vi "FormCalibra10-joao.vi"() -> ()   [LabVIEW 2014]
uses:
  testMachine.ctl
  mainMachine.ctl
  <vilib>/Instr/_visa.llb/VISA Configure Serial Port (Instr).vi
  <vilib>/express/express shared/transition.llb/Dynamic To Waveform Array.vi
  <vilib>/express/express signal manip/GetorSetDDTAttributes/Set DDT Attributes/SetT0.vi
  <vilib>/express/express shared/transition.llb/Waveform Array To Dynamic.vi
  <vilib>/express/express signal manip/GetorSetDDTAttributes/Set DDT Attributes/Set DDT Properties.xnode
panel:
  in  "editSpeedOffset":dbl caption="Offset (Km/h)"
  in  "editSetTempRefB":dbl caption="Offset B" step=0.01 format="%#_2f"
  in  "VISA Serial Port":refnum<visa-resource-name>
  in  "Lower level":dbl
  in  "hysteresis":dbl format="%.2p"
  in  "level":dbl format="%.2p"
  out "rpm":bool
  out "editTotalWaitLimit":u8
  out "editCountWaitLimit":u8
  out "ledWaitState":bool caption="Wait State"
  out "sliderWaitUpperTime":u8(slide) max=50 scale=0.0..100.0
  out "slideWaitLowerTime":u8(slide) max=30 scale=0.0..100.0
  out "slideWaitTime":u8(slide) scale=0.0..100.0
  out "labelTestTime":string caption="Tempo total de ensaio"
  in  "editSetWaitTime":u8 caption="Interval between snubs (s)" step=1 format="%0d"
  in  "stop":bool
  out "ledAcquireState":bool caption="Acquire State"
  out "editTotalLowerLimit":u8
  out "editCountLowerLimit":u8
  out "editTotalUpperLimit":u8
  out "editCountUpperLimit":u8
  out "ledEnsaio 3":bool
  out "ledBrakeState":bool caption="Brake State"
  out "ledExitState":bool caption="Exit State"
  out "ledMotorState":bool caption="Motor State"
  out "ledInit2State":bool caption="Init State"
  out "ledBlockState":bool caption="Block State"
  out "ledRunningState":bool caption="Running State"
  out "ledReadyState":bool caption="Ready State"
  out "ledInitState":bool caption="Init State"
  out "mainMachine":T1
  out "testMachine":T2=enum."finish"
  in  "editSetPathToFile":path
  in  "buttonStop":bool
  in  "buttonStart":bool
  out "graphForce":dynamicdata(graph)
  in  "editOffsetForce":dbl caption="Tare (KN)" min=-100.0 max=100.0 step=0.1
  in  "editSetForce":dbl=0.1 caption="Conversion Factor" min=0.1 max=100.0 step=0.1
  out "editForce":dbl caption="Force (KN)" format="%#_4f"
  out "graphSpeed":dynamicdata(graph)
  in  "editSetSpeed":dbl caption="Conversion Factor"
  out "editSpeed":dbl caption="Speed (km/h)" format="%#_4f"
  out "editEngineSpeed":dbl caption="Frequency (Hz)" format="%#_4f"
  in  "editSetWaitLowerTime":u8 caption="Lower Wait Interval (s)"
  in  "editSetWaitUpperTime":u8=3 caption="Upper Wait Interval (s)"
  in  "editSetNumberOfCycles":u16 caption="Number of snubs" max=999 step=1 format="%0d"
  in  "editSetLowerLimit":u32 caption="Lower Limit (km/h)"
  in  "editSetUpperLimit":u32 caption="Upper Limit (km/h)"
  out "editTempB":dbl caption="Temperature B (ºC)"
  out "editTempA":dbl caption="Temperature A (ºC)"
  in  "editSetTempRefA":dbl caption="Offset A" step=0.01 format="%#_2f"
  out "ledMotor":bool
  out "ledBrake":bool
  out "ledEnsaio":bool
  out "labelTotalCycle":string
  out "labelCurrentCycle":string
  out "labelSystemTitle":string
  in  "editCurrCycleCtr":u32
  in  "velocidade 2":u32
  out "velocidade":u32
  # "Brake Test Bench"
  # "Com Port"
  # "Temperature"
  # "Rotation"
  # "Load Cell"
  # "Test Configuration"
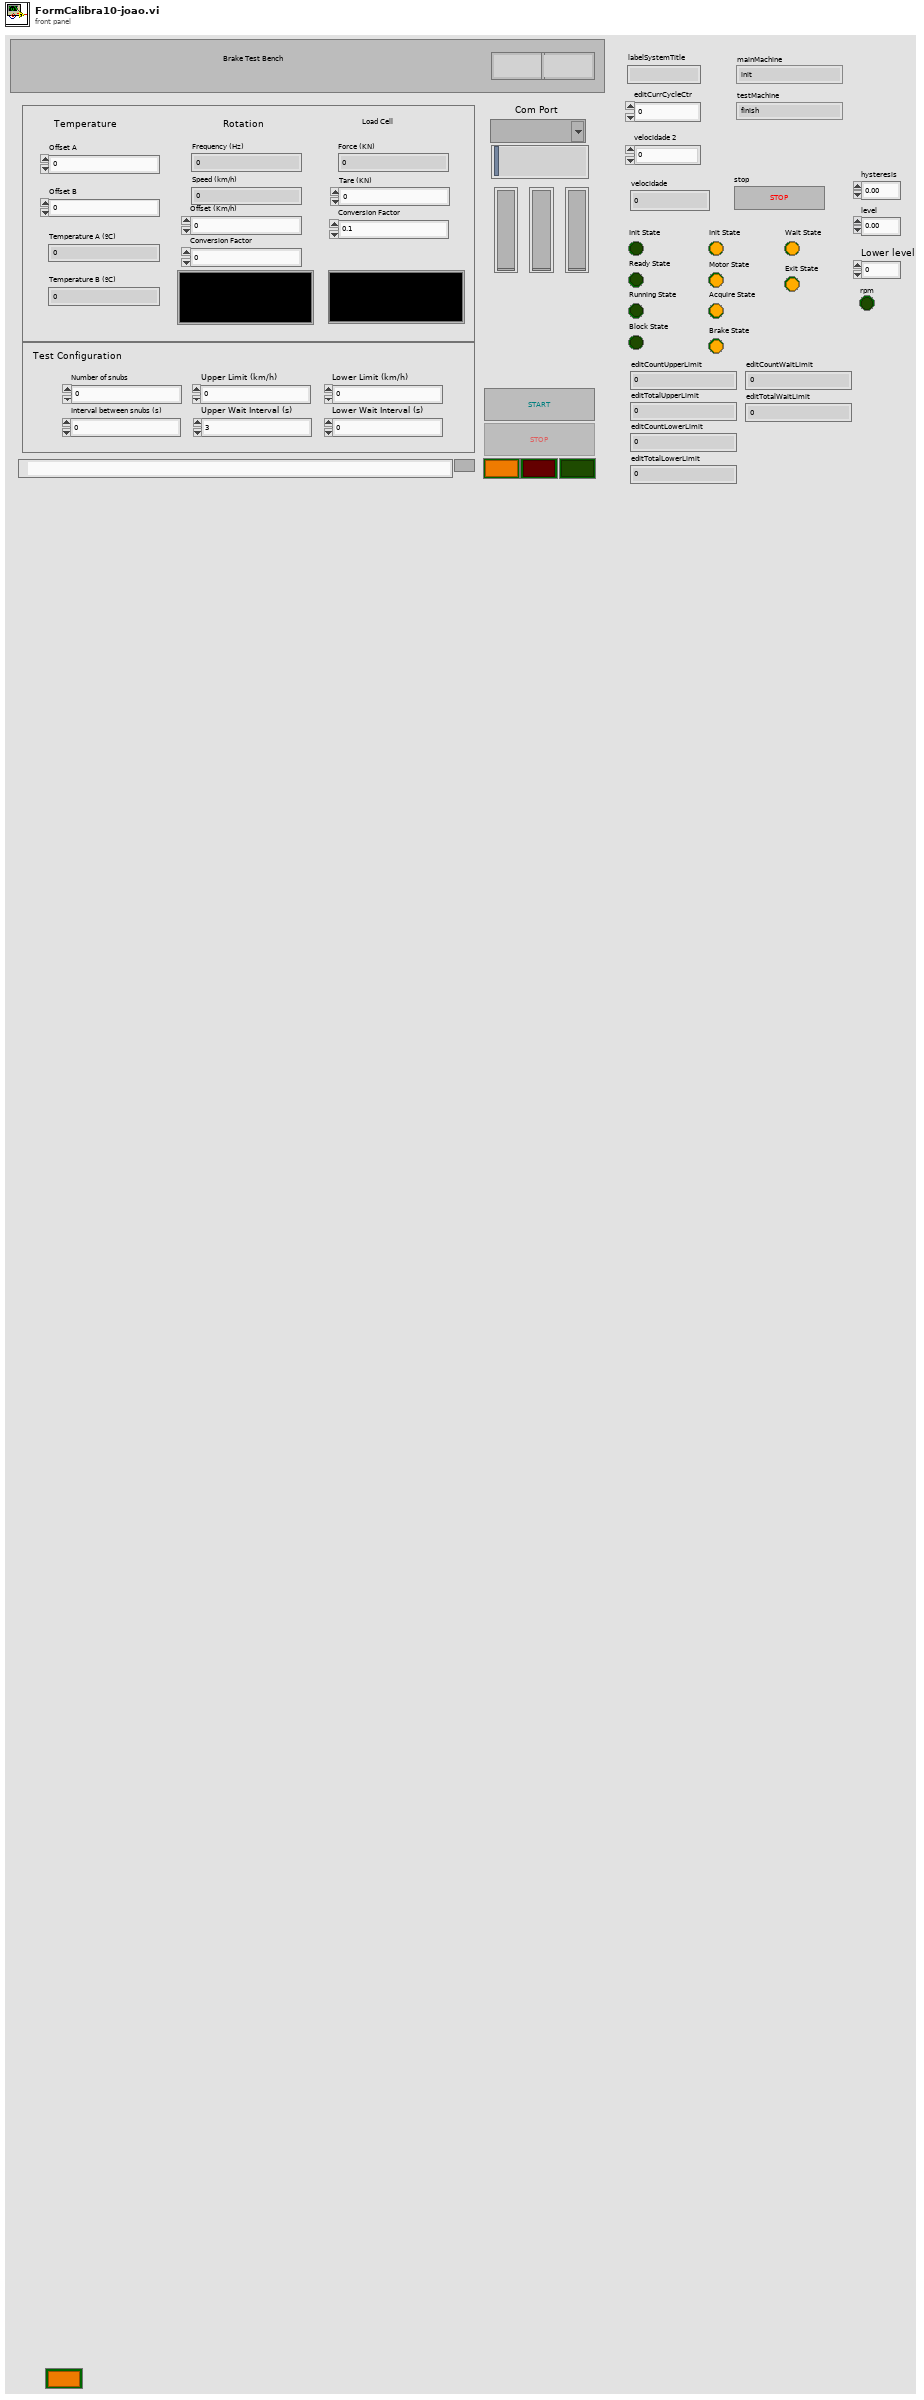
[diagram p1: front panel]
types:
  T1 = typedef "mainMachine.ctl" = enum16{"init", "ready", "running", "blocked", "finish"}
  T2 = typedef "testMachine.ctl" = enum16{"init", "motor", "motor acquire", "brake", "brake acquire", "wait ", "finish", "exit"}
  T3 = enum8{"Enabled", "Disabled", "Disabled and Grayed Out"}
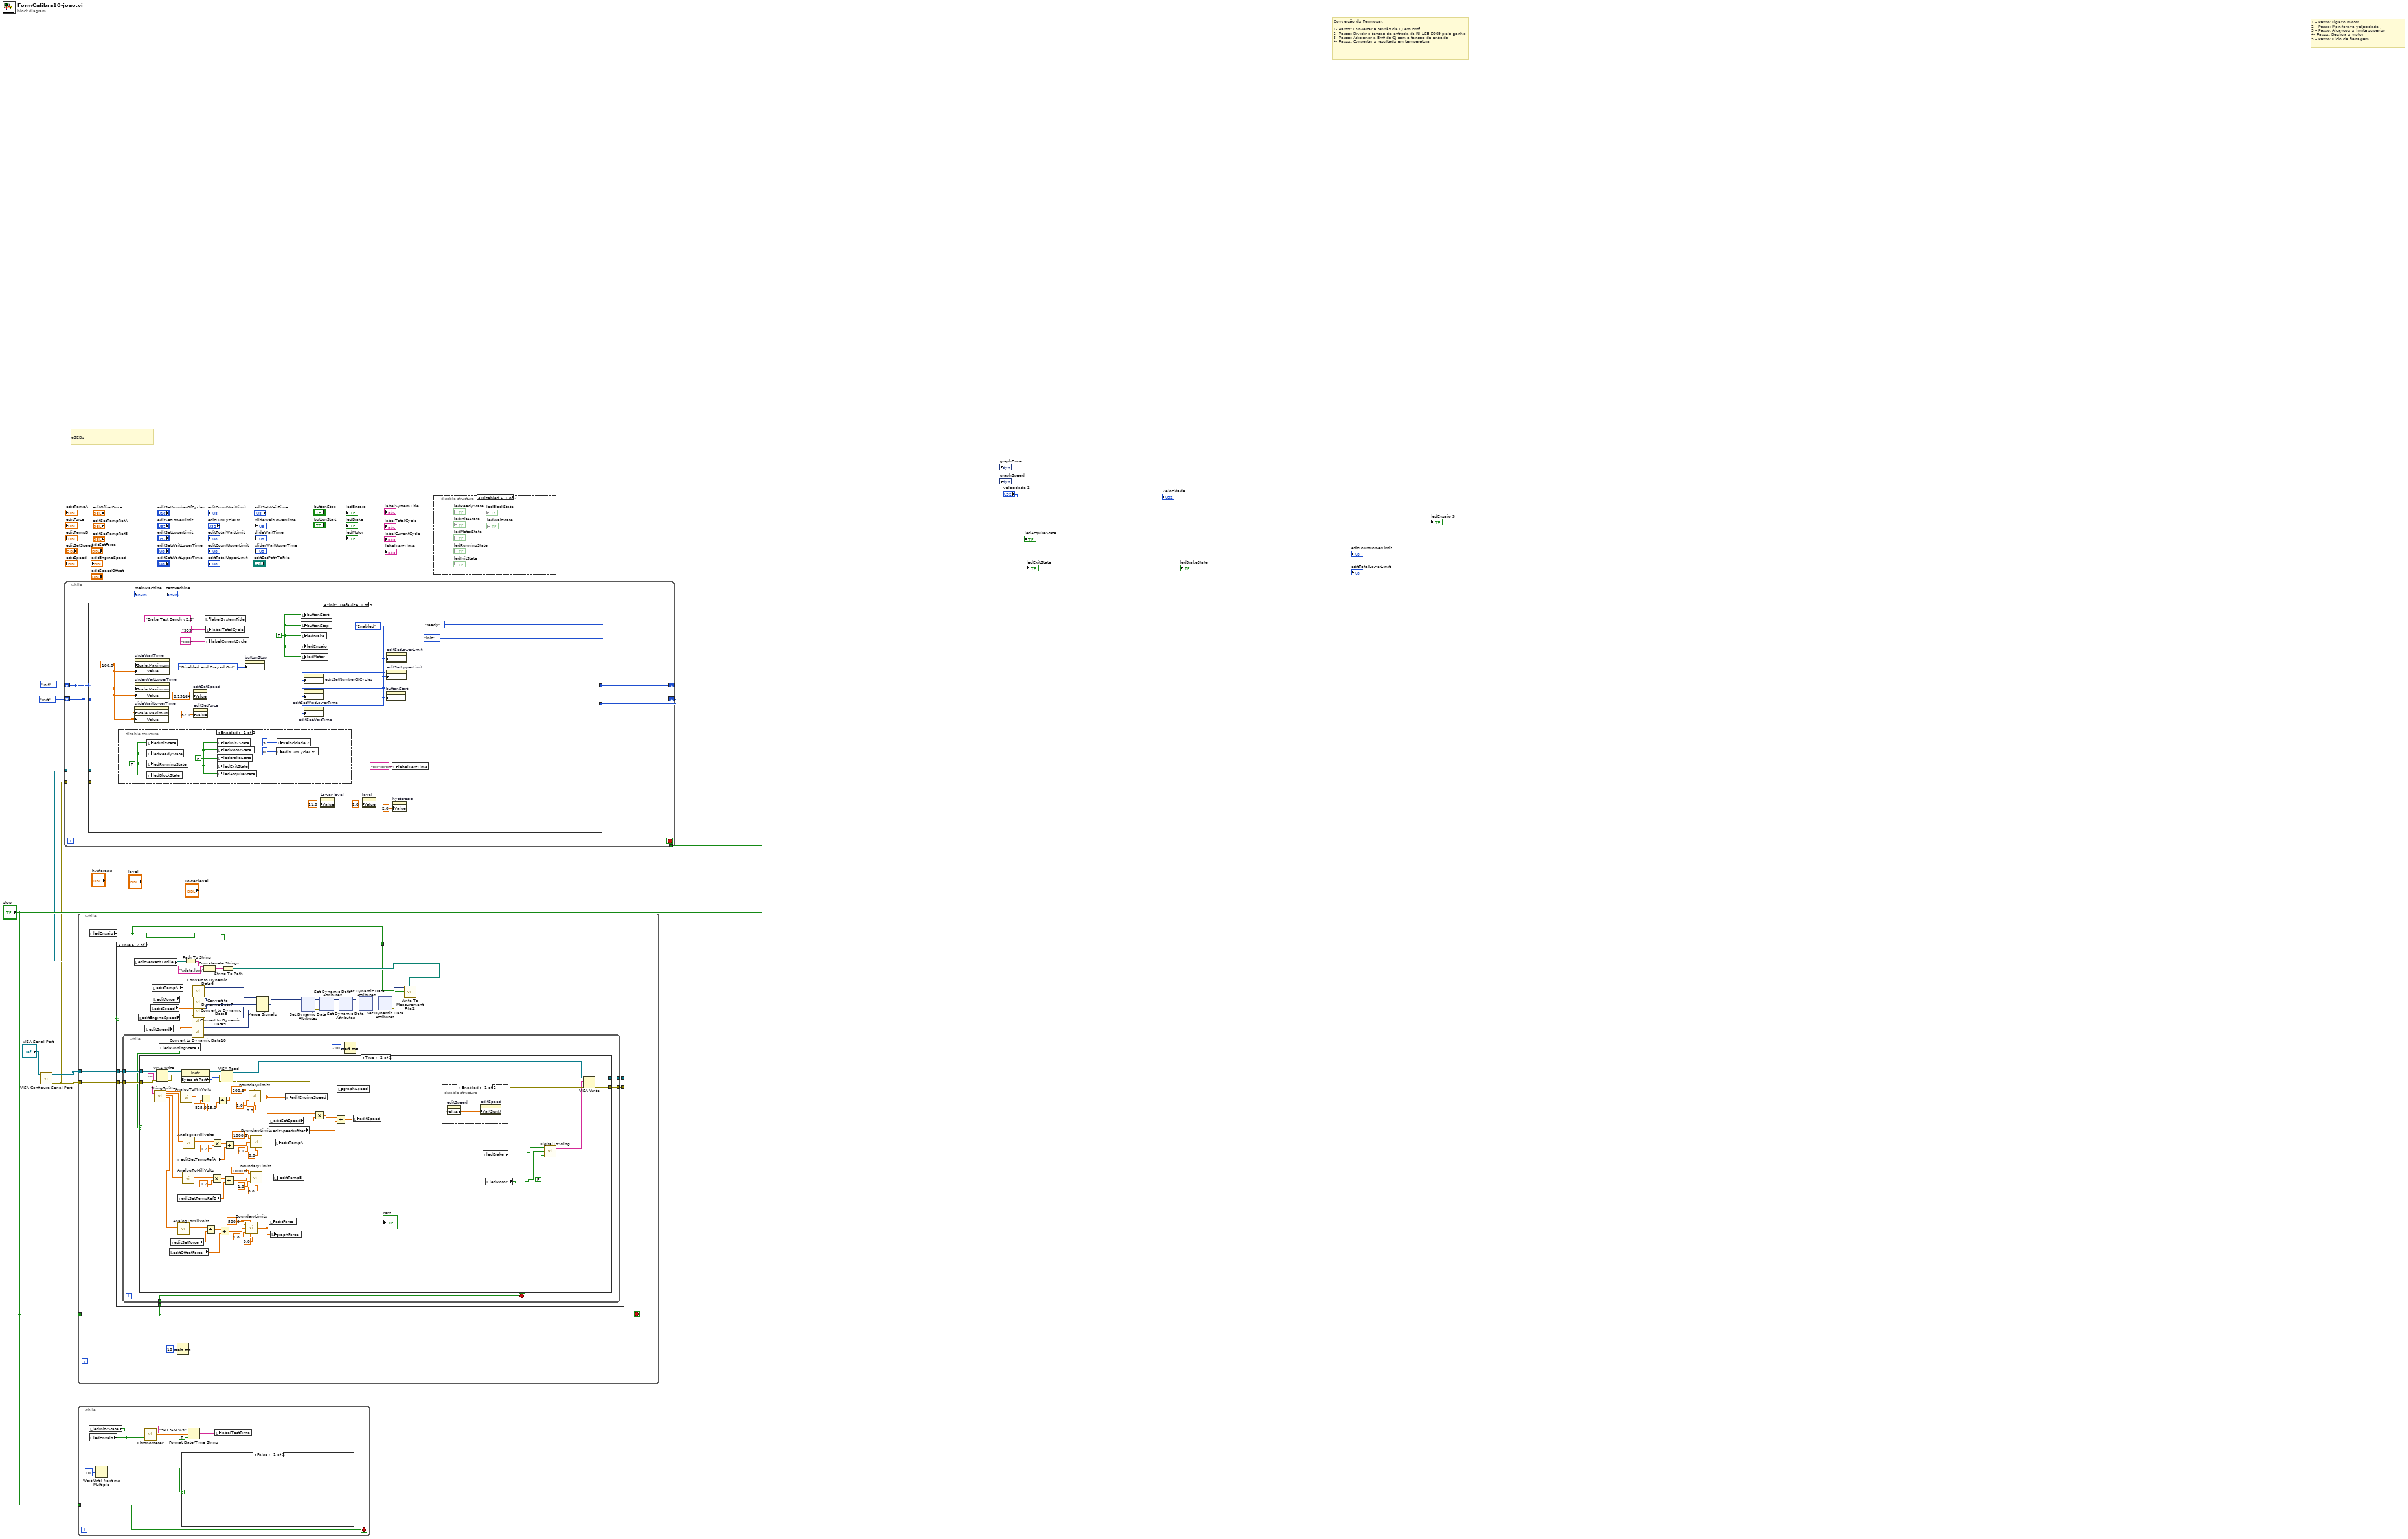
[diagram p0: block diagram]
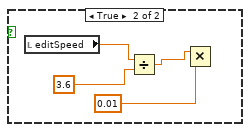
[diagram p3: hidden frame]
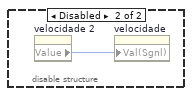
[diagram p6: hidden frame]
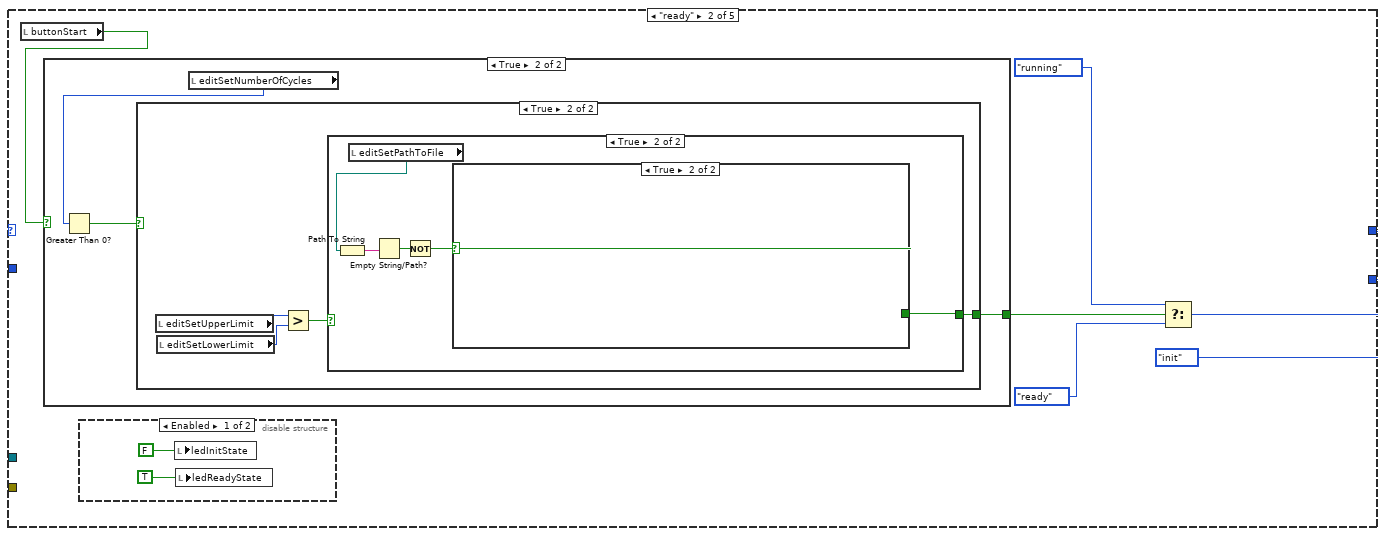
[diagram p8: hidden frame]
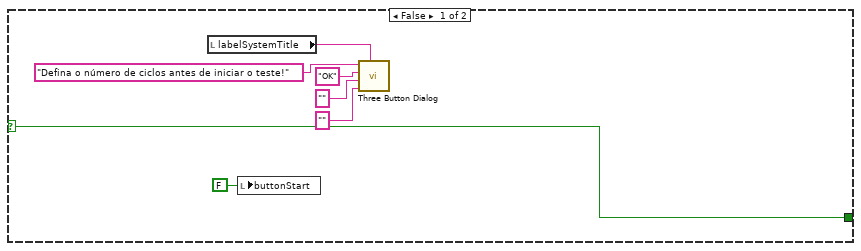
[diagram p11: hidden frame]
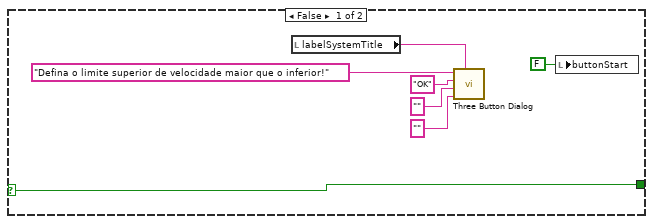
[diagram p12: hidden frame]
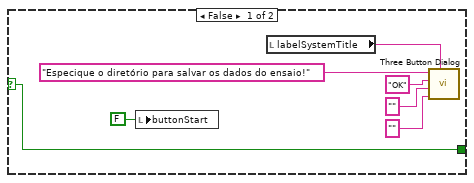
[diagram p13: hidden frame]
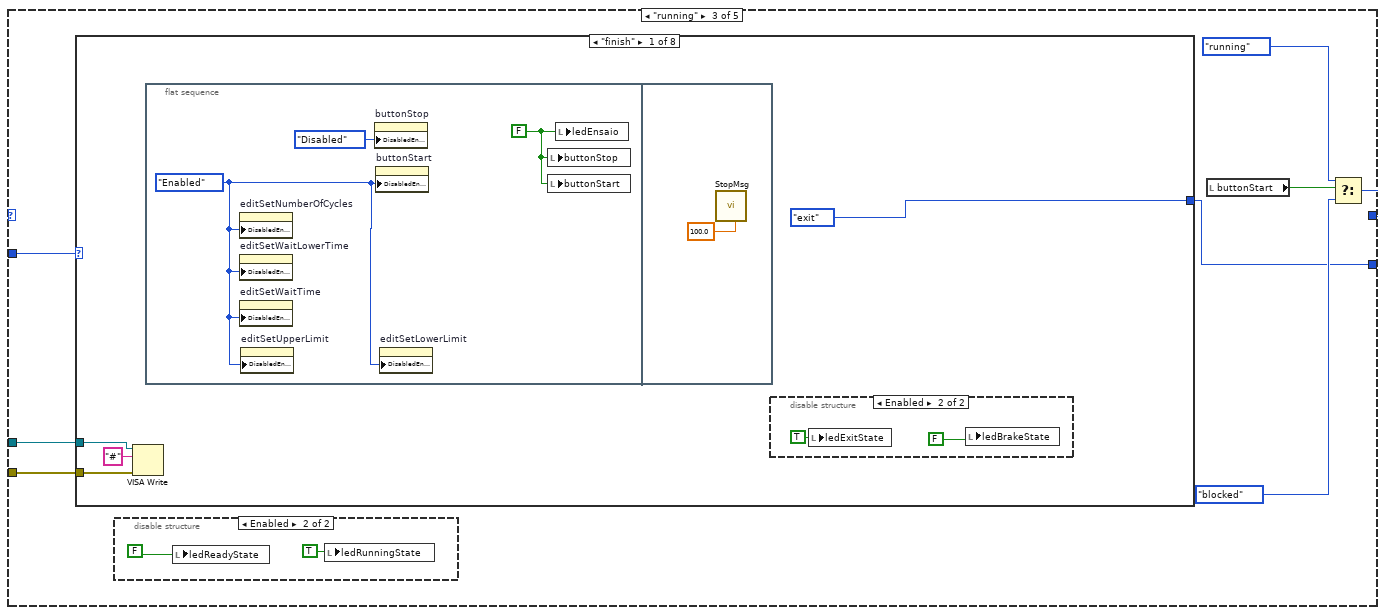
[diagram p14: hidden frame]
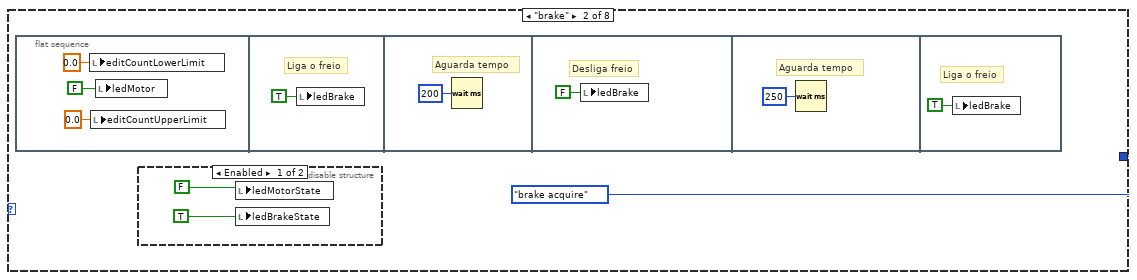
[diagram p17: hidden frame]
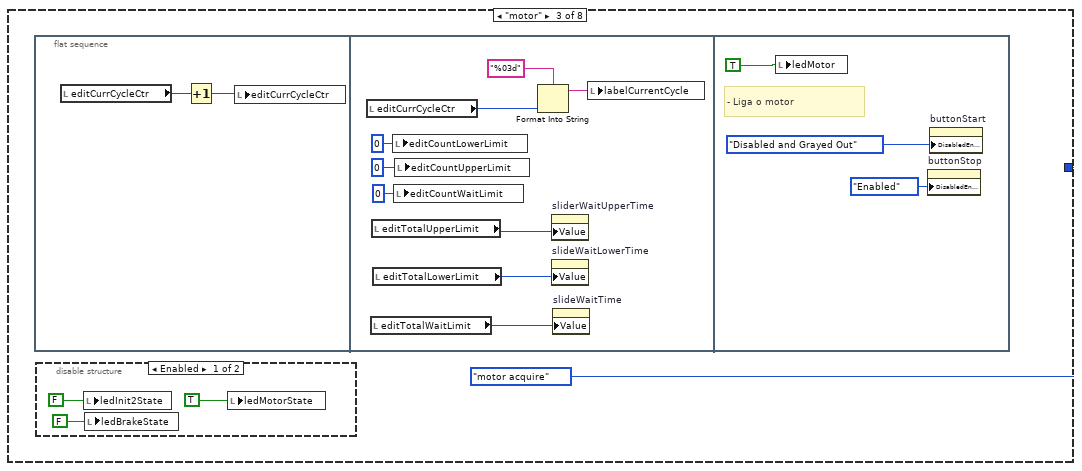
[diagram p19: hidden frame]
diagram:
  # "eSEDs"
  # "1 - Passo: Ligar o motor\n2 - Passo: Monitorar a velocidade\n3 - Passo: Alcancou o limite superior\n4- Passo: Desliga o motor\n5 - Passo: Ciclo de frenagem"
  # "Conversão do Termopar:\n\n1- Passo: Converter a tensão da CJ em Emf\n2- Passo: Dividir a tensão de entrada da NI USB 6009 pelo ganho\n3- Passo: Adicionar a Emf da CJ com a tensão de entrada\n4- Passo: Converter o resultado em temperatura"
  n1 = call-poly "VISA Configure Serial Port"("VISA resource name"="VISA Serial Port") -> ("VISA resource name out"=w3:refnum<visa-resource-name>, "error out"=w2:errorcluster)  [unwired: 13 in]
  n2 = while {
    shift-right: [w14] -> _
    shift-left: mainMachine."init" ("mainMachine") -> [w11]
    shift-right: [w13] -> _
    shift-left: testMachine."init" ("testMachine") -> [w12]
    tunnel: "stop" -> [w10]
    tunnel: w3 -> [w9]
    tunnel: w2 -> [w8]
    stop <- w10 stop-if-true
    n3 = case shown="\"init\", Default" w11 {
      tunnel: [mainMachine."ready" ("mainMachine") w34 w81 w230 mainMachine."finish" ("mainMachine")] -> w14
      tunnel: [testMachine."init" ("testMachine") testMachine."init" ("testMachine") w80 testMachine."init" ("testMachine") testMachine."init" ("testMachine")] -> w13
      tunnel: w12 -> [_ _ w79 _ _]
      tunnel: w9 -> [_ _ w78 _ _]
      tunnel: w8 -> [_ _ w77 _ _]
      frame "init", Default {
        w21 = 100.0 ("Scale.Range:Maximum")
        w22 = T3."Enabled" ("Disabled")
        w28 = FALSE ("motor")
        n4 = disable-structure shown="Enabled" {
          frame Enabled {
            w30 = FALSE
            w31 = FALSE
            n5 = local write "ledInitState"(w31) -> ()
            n6 = local write "ledReadyState"(w31) -> ()
            n7 = local write "ledRunningState"(w31) -> ()
            n8 = local write "ledBlockState"(w31) -> ()
            n9 = local write "ledInit2State"(w30) -> ()
            n10 = local write "ledMotorState"(w30) -> ()
            n11 = local write "ledBrakeState"(w30) -> ()
            n12 = local write "ledExitState"(w30) -> ()
            n13 = local write "ledAcquireState"(w30) -> ()
            n14 = local write "editCurrCycleCtr"(u32 0 ("currentCycleCtr")) -> ()
            n15 = local write "velocidade 2"(u32 5 ("velocidade 2")) -> ()
          }
          frame Disabled {
          }
        }
        n16 = property on="slideWaitLowerTime" class="Slide (strict)"("Scale.Maximum"=w21, "Value"=w21) -> ()  [unwired: 2 in, 2 out]
        n17 = property on="slideWaitTime" class="Slide (strict)"("Scale.Maximum"=w21, "Value"=w21) -> ()  [unwired: 2 in, 2 out]
        n18 = property on="sliderWaitUpperTime" class="Slide (strict)"("Scale.Maximum"=w21, "Value"=w21) -> ()  [unwired: 2 in, 2 out]
        n19 = property on="editSetSpeed" class="DigNum (strict)"("Value"=0.15164 ("editSetSpeed")) -> ()  [unwired: 2 in, 2 out]
        n20 = property on="editSetForce" class="DigNum (strict)"("Value"=82.0 ("editSetForce")) -> ()  [unwired: 2 in, 2 out]
        n21 = local write "labelSystemTitle"("Brake Test Bench v2.0" ("systemTitle")) -> ()
        n22 = local write "labelCurrentCycle"("000" ("currentCycle")) -> ()
        n23 = local write "labelTotalCycle"("999" ("totalCycle")) -> ()
        n24 = property on="buttonStop" class="Bool (strict)"("DisabledEnum"=T3."Disabled and Grayed Out" ("Disabled")) -> ()  [unwired: 2 in, 2 out]
        n25 = local write "buttonStart"(w28) -> ()
        n26 = local write "buttonStop"(w28) -> ()
        n27 = local write "ledBrake"(w28) -> ()
        n28 = local write "ledEnsaio"(w28) -> ()
        n29 = local write "ledMotor"(w28) -> ()
        n30 = property on="editSetNumberOfCycles" class="DigNum (strict)"("DisabledEnum"=w22) -> ()  [unwired: 2 in, 2 out]
        n31 = property on="editSetWaitLowerTime" class="DigNum (strict)"("DisabledEnum"=w22) -> ()  [unwired: 2 in, 2 out]
        n32 = property on="editSetWaitTime" class="DigNum (strict)"("DisabledEnum"=w22) -> ()  [unwired: 2 in, 2 out]
        n33 = property on="Lower level" class="DigNum (strict)"("Value"=11.0 ("Lower level")) -> ()  [unwired: 2 in, 2 out]
        n34 = property on="level" class="DigNum (strict)"("Value"=2.0 ("level")) -> ()  [unwired: 2 in, 2 out]
        n35 = property on="buttonStart" class="Bool (strict)"("DisabledEnum"=w22) -> ()  [unwired: 2 in, 2 out]
        n36 = property on="editSetLowerLimit" class="DigNum (strict)"("DisabledEnum"=w22) -> ()  [unwired: 2 in, 2 out]
        n37 = property on="editSetUpperLimit" class="DigNum (strict)"("DisabledEnum"=w22) -> ()  [unwired: 2 in, 2 out]
        n38 = local write "labelTestTime"("00:00:00" ("labelTestTime")) -> ()
        n39 = property on="hysteresis" class="DigNum (strict)"("Value"=2.0 ("hysteresis")) -> ()  [unwired: 2 in, 2 out]
      }
      frame "ready" {
        n40 = local read "buttonStart"() -> (w37:bool)
        n41 = case shown="True" w37 {
          selector: w37 -> [w42 _]
          tunnel: [w42 w43] -> w36
          frame False {
          }
          frame True {
            n42 = local read "editSetNumberOfCycles"() -> (w44:u16)
            n43 = Greater Than 0?(x=w44) -> (x > 0?=w45:bool)
            n44 = case shown="True" w45 {
              selector: w45 -> [w52 _]
              tunnel: [w52 w53] -> w43
              frame False {
                n45 = local read "labelSystemTitle"() -> (w47:string)
                n46 = local write "buttonStart"(FALSE ("startButton")) -> ()
                n47 = call <vilib>:"Three Button Dialog.vi"("Window Title (\"\")"=w47, "Right Button Text (\"Cancel\")"="" ("Right Button Text (\"Cancel\")"), "Center Button Text (\"No\")"="" ("Center Button Text (\"No\")"), "Left Button Text (\"Yes\")"="OK" ("Left Button Text (\"Yes\")"), "message"="Defina o número de ciclos antes de iniciar o teste!") -> ()  [unwired: 6 in, 1 out]
              }
              frame True {
                n48 = local read "editSetUpperLimit"() -> (w55:u32)
                n49 = local read "editSetLowerLimit"() -> (w54:u32)
                n50 = Greater?(x=w55, y=w54) -> (0:w56:bool)
                n51 = case shown="True" w56 {
                  selector: w56 -> [w63 _]
                  tunnel: [w63 w66] -> w53
                  frame False {
                    n52 = local read "labelSystemTitle"() -> (w58:string)
                    n53 = call <vilib>:"Three Button Dialog.vi"("Window Title (\"\")"=w58, "Right Button Text (\"Cancel\")"="" ("Right Button Text (\"Cancel\")"), "Center Button Text (\"No\")"="" ("Center Button Text (\"No\")"), "Left Button Text (\"Yes\")"="OK" ("Left Button Text (\"Yes\")"), "message"="Defina o limite superior de velocidade maior que o inferior!") -> ()  [unwired: 6 in, 1 out]
                    n54 = local write "buttonStart"(FALSE ("startButton")) -> ()
                  }
                  frame True {
                    n55 = local read "editSetPathToFile"() -> (w68:path)
                    n56 = Path To String(path=w68) -> (string=w67:string)
                    n57 = Empty String/Path?(string/path=w67) -> (empty?=w65:bool)
                    n58 = Not(x=w65) -> (.not. x?=w64:bool)
                    n59 = case shown="True" w64 {
                      selector: w64 -> [w75 w76]
                      tunnel: [w75 w76] -> w66
                      frame False {
                        n60 = local write "buttonStart"(FALSE ("startButton")) -> ()
                        n61 = local read "labelSystemTitle"() -> (w70:string)
                        n62 = call <vilib>:"Three Button Dialog.vi"("Window Title (\"\")"=w70, "Right Button Text (\"Cancel\")"="" ("Right Button Text (\"Cancel\")"), "Center Button Text (\"No\")"="" ("Center Button Text (\"No\")"), "Left Button Text (\"Yes\")"="OK" ("Left Button Text (\"Yes\")"), "message"="Especique o diretório para salvar os dados do ensaio!") -> ()  [unwired: 6 in, 1 out]
                      }
                      frame True {
                      }
                    }
                  }
                }
              }
            }
          }
        }
        n63 = disable-structure shown="Enabled" {
          frame Enabled {
            n64 = local write "ledInitState"(FALSE ("ledReady")) -> ()
            n65 = local write "ledReadyState"(TRUE ("ledReady")) -> ()
          }
          frame Disabled {
          }
        }
        n66 = Select(t=mainMachine."running" ("mainMachine"), s=w36, f=mainMachine."ready" ("mainMachine")) -> (s? t:f=w34:T1)
      }
      frame "running" {
        n67 = case shown="\"finish\"" w79 {
          tunnel: [testMachine."exit" ("testMachine") testMachine."brake acquire" ("testMachine") testMachine."motor acquire" ("testMachine") testMachine."motor" ("testMachine") w160 w180 testMachine."exit" ("testMachine") w213] -> w80
          tunnel: w78 -> [w88 _ _ w127 _ _ _ _]
          tunnel: w77 -> [w87 _ _ w126 _ _ _ _]
          frame "finish" {
            n68 = VISA Write(VISA resource name=w88, write buffer="#", error in (no error)=w87) -> ()  [unwired: 3 out]
            n69 = flat-sequence {
              frame #0 {
                w94 = FALSE ("ledReady")
                w93 = T3."Enabled" ("Disabled")
                n70 = property on="editSetNumberOfCycles" class="DigNum (strict)"("DisabledEnum"=w93) -> ()  [unwired: 2 in, 2 out]
                n71 = property on="editSetWaitLowerTime" class="DigNum (strict)"("DisabledEnum"=w93) -> ()  [unwired: 2 in, 2 out]
                n72 = property on="editSetWaitTime" class="DigNum (strict)"("DisabledEnum"=w93) -> ()  [unwired: 2 in, 2 out]
                n73 = property on="editSetUpperLimit" class="DigNum (strict)"("DisabledEnum"=w93) -> ()  [unwired: 2 in, 2 out]
                n74 = property on="buttonStop" class="Bool (strict)"("DisabledEnum"=T3."Disabled" ("Disabled")) -> ()  [unwired: 2 in, 2 out]
                n75 = property on="buttonStart" class="Bool (strict)"("DisabledEnum"=w93) -> ()  [unwired: 2 in, 2 out]
                n76 = property on="editSetLowerLimit" class="DigNum (strict)"("DisabledEnum"=w93) -> ()  [unwired: 2 in, 2 out]
                n77 = local write "buttonStop"(w94) -> ()
                n78 = local write "buttonStart"(w94) -> ()
                n79 = local write "ledEnsaio"(w94) -> ()
              }
              frame #1 {
                n80 = call "StopMsg.vi"("Max Value (100)"=100.0) -> ()  [unwired: 8 in, 2 out]
              }
            }
            n81 = disable-structure shown="Enabled" {
              frame Disabled {
              }
              frame Enabled {
                n82 = local write "ledExitState"(TRUE ("ledReady")) -> ()
                n83 = local write "ledBrakeState"(FALSE ("ledReady")) -> ()
              }
            }
          }
          frame "brake" {
            n84 = flat-sequence {
              frame #0 {
                n85 = local write "editCountLowerLimit"(0.0 ("editCountUpperLimit")) -> ()
                n86 = local write "editCountUpperLimit"(0.0 ("editCountUpperLimit")) -> ()
                n87 = local write "ledMotor"(FALSE ("motor")) -> ()
              }
              frame #1 {
                # "Liga o freio"
                n88 = local write "ledBrake"(TRUE ("freio")) -> ()
              }
              frame #2 {
                # "Aguarda tempo"
                n89 = Wait (ms)(milliseconds to wait=u32 200) -> ()  [unwired: 1 out]
              }
              frame #3 {
                # "Desliga freio"
                n90 = local write "ledBrake"(FALSE ("freio")) -> ()
              }
              frame #4 {
                # "Aguarda tempo"
                n91 = Wait (ms)(milliseconds to wait=u32 250) -> ()  [unwired: 1 out]
              }
              frame #5 {
                # "Liga o freio"
                n92 = local write "ledBrake"(TRUE ("freio")) -> ()
              }
            }
            n93 = disable-structure shown="Enabled" {
              frame Enabled {
                n94 = local write "ledMotorState"(FALSE ("ledReady")) -> ()
                n95 = local write "ledBrakeState"(TRUE ("ledReady")) -> ()
              }
              frame Disabled {
              }
            }
          }
          frame "motor" {
            n96 = flat-sequence {
              frame #0 {
                n97 = local read "editCurrCycleCtr"() -> (w113:u32)
                n98 = Increment(x=w113) -> (x+1=w112:u32)
                n99 = local write "editCurrCycleCtr"(w112) -> ()
              }
              frame #1 {
                n100 = local read "editCurrCycleCtr"() -> (w120:u32)
                n101 = local read "editTotalWaitLimit"() -> (w114:u8)
                n102 = local read "editTotalUpperLimit"() -> (w116:u8)
                n103 = local read "editTotalLowerLimit"() -> (w115:u8)
                n104 = local write "editCountLowerLimit"(u8 0 ("editCountLowerLimit")) -> ()
                n105 = local write "editCountWaitLimit"(u8 0 ("editCountWaitLimit")) -> ()
                n106 = local write "editCountUpperLimit"(u8 0 ("editCountUpperLimit")) -> ()
                n107 = Format Into String(format string="%03d", w120) -> (resulting string=w121:string)  [unwired: 2 in, 1 out]
                n108 = property on="sliderWaitUpperTime" class="Slide (strict)"("Value"=w116) -> ()  [unwired: 2 in, 2 out]
                n109 = property on="slideWaitLowerTime" class="Slide (strict)"("Value"=w115) -> ()  [unwired: 2 in, 2 out]
                n110 = property on="slideWaitTime" class="Slide (strict)"("Value"=w114) -> ()  [unwired: 2 in, 2 out]
                n111 = local write "labelCurrentCycle"(w121) -> ()
              }
              frame #2 {
                # "- Liga o motor"
                n112 = local write "ledMotor"(TRUE ("motor")) -> ()
                n113 = property on="buttonStop" class="Bool (strict)"("DisabledEnum"=T3."Enabled" ("Disabled")) -> ()  [unwired: 2 in, 2 out]
                n114 = property on="buttonStart" class="Bool (strict)"("DisabledEnum"=T3."Disabled and Grayed Out" ("Disabled")) -> ()  [unwired: 2 in, 2 out]
              }
            }
            n115 = disable-structure shown="Enabled" {
              frame Enabled {
                n116 = local write "ledInit2State"(FALSE ("ledReady")) -> ()
                n117 = local write "ledBrakeState"(FALSE ("ledReady")) -> ()
                n118 = local write "ledMotorState"(TRUE ("ledReady")) -> ()
              }
              frame Disabled {
              }
            }
          }
          frame "init", Default {
            n119 = stacked-sequence {
              tunnel: w127 -> [_ _ _]
              tunnel: w126 -> [_ _ _]
              frame #0 {
                w135 = FALSE ("ensaio")
                n120 = local write "ledMotor"(w135) -> ()
                n121 = local write "ledBrake"(w135) -> ()
                n122 = local read "editSetNumberOfCycles"() -> (w142:u16)
                n123 = local read "editSetWaitLowerTime"() -> (w136:u8)
                n124 = local read "editSetWaitUpperTime"() -> (w139:u8)
                n125 = local read "editSetWaitTime"() -> (w130:u8)
                n126 = Multiply(x=w130, y=u32 10) -> (x*y=w131:u32)
                n127 = Multiply(x=w136, y=u32 10) -> (x*y=w134:u32)
                n128 = Format Into String(format string="%03d", w142) -> (resulting string=w143:string)  [unwired: 2 in, 1 out]
                n129 = Multiply(x=w139, y=u32 10) -> (x*y=w133:u32)
                n130 = local write "editTotalLowerLimit"(w134) -> ()
                n131 = local write "editTotalUpperLimit"(w133) -> ()
                n132 = local write "editTotalWaitLimit"(w131) -> ()
                n133 = local write "labelTotalCycle"(w143) -> ()
                n134 = local write "editCurrCycleCtr"(u32 0 ("currentCycleCtr")) -> ()
                n135 = local write "labelCurrentCycle"("000" ("currentCycle")) -> ()
              }
              frame #1 {
                w151 = T3."Disabled" ("Disabled")
                n136 = property on="editSetNumberOfCycles" class="DigNum (strict)"("DisabledEnum"=w151) -> ()  [unwired: 2 in, 2 out]
                n137 = property on="editSetWaitLowerTime" class="DigNum (strict)"("DisabledEnum"=w151) -> ()  [unwired: 2 in, 2 out]
                n138 = property on="editSetWaitTime" class="DigNum (strict)"("DisabledEnum"=w151) -> ()  [unwired: 2 in, 2 out]
                n139 = local read "editTotalUpperLimit"() -> (w154:u8)
                n140 = property on="sliderWaitUpperTime" class="Slide (strict)"("Scale.Maximum"=w154, "Scale.Minimum"=0.0 ("Scale.Range:Minimum"), "Scale.Increment"=1.0 ("Scale.Range:Increment"), "Value"=w154) -> ()  [unwired: 2 in, 2 out]
                n141 = local read "editTotalLowerLimit"() -> (w148:u8)
                n142 = property on="slideWaitLowerTime" class="Slide (strict)"("Scale.Maximum"=w148, "Scale.Minimum"=0.0 ("Scale.Range:Minimum"), "Scale.Increment"=1.0 ("Scale.Range:Increment"), "Value"=w148) -> ()  [unwired: 2 in, 2 out]
                n143 = local read "editTotalWaitLimit"() -> (w145:u8)
                n144 = property on="slideWaitTime" class="Slide (strict)"("Scale.Maximum"=w145, "Scale.Minimum"=0.0 ("Scale.Range:Minimum"), "Scale.Increment"=1.0 ("Scale.Range:Increment"), "Value"=w145) -> ()  [unwired: 2 in, 2 out]
                n145 = call "StarMsg.vi"("Show"=TRUE, "Max Value (100)"=100.0) -> ()  [unwired: 7 in, 2 out]
                n146 = property on="editSetLowerLimit" class="DigNum (strict)"("DisabledEnum"=w151) -> ()  [unwired: 2 in, 2 out]
                n147 = property on="editSetUpperLimit" class="DigNum (strict)"("DisabledEnum"=w151) -> ()  [unwired: 2 in, 2 out]
              }
              frame #2 {
                n148 = local write "ledEnsaio"(TRUE ("ensaio")) -> ()
              }
            }
            n149 = disable-structure shown="Enabled" {
              frame Enabled {
                n150 = local write "ledInit2State"(TRUE ("ledReady")) -> ()
              }
              frame Disabled {
              }
            }
          }
          frame "motor acquire" {
            n151 = disable-structure shown="Enabled" {
              frame Enabled {
                n152 = local read "ledAcquireState"() -> (w169:bool)
                n153 = Not(x=w169) -> (.not. x?=w168:bool)
                n154 = local write "ledAcquireState"(w168) -> ()
              }
              frame Disabled {
              }
            }
            n155 = Wait (ms)(milliseconds to wait=u32 100) -> ()  [unwired: 1 out]
            n156 = disable-structure shown="Enabled" {
              disable-tunnel: [w166 w167] -> w159
              frame Enabled {
                n157 = property on="editSpeed" class="DigNum (strict)"() -> ("Value"=w166:dbl)  [unwired: 2 in, 2 out]
              }
              frame Disabled {
                n158 = property on="velocidade" class="DigNum (strict)"() -> ("Value"=w167:u32)  [unwired: 2 in, 2 out]
              }
            }
            n159 = property on="editSetUpperLimit" class="DigNum (strict)"() -> ("Value"=w158:u32)  [unwired: 2 in, 2 out]
            n160 = Greater Or Equal?(x=w159, y=w158) -> (x >= y?=w164:bool)
            n161 = case shown="True" w164 {
              selector: w164 -> [w170 _]
              tunnel: [w170 w171] -> w163
              frame False {
              }
              frame True {
                n162 = flat-sequence {
                  tunnel: [w176] -> w171
                  frame #0 {
                    n163 = local read "editCountUpperLimit"() -> (w174:u8)
                    n164 = Increment(x=w174) -> (x+1=w172:u8)
                    n165 = local write "editCountUpperLimit"(w172) -> ()
                    n166 = local read "editTotalUpperLimit"() -> (w173:u8)
                    n167 = Subtract(x=w173, y=w172) -> (x-y=w175:u8)
                    n168 = property on="sliderWaitUpperTime" class="Slide (strict)"("Value"=w175) -> ()  [unwired: 2 in, 2 out]
                  }
                  frame #1 {
                    n169 = local read "editCountUpperLimit"() -> (w178:u8)
                    n170 = local read "editTotalUpperLimit"() -> (w177:u8)
                    n171 = Greater Or Equal?(x=w178, y=w177) -> (x >= y?=w176:bool)
                  }
                }
              }
            }
            n172 = Select(t=testMachine."brake" ("testMachine"), s=w163, f=testMachine."motor acquire" ("testMachine")) -> (s? t:f=w160:T2)
          }
          frame "brake acquire" {
            n173 = disable-structure shown="Enabled" {
              frame Enabled {
                n174 = local read "ledAcquireState"() -> (w188:bool)
                n175 = Not(x=w188) -> (.not. x?=w187:bool)
                n176 = local write "ledAcquireState"(w187) -> ()
              }
              frame Disabled {
              }
            }
            n177 = Wait (ms)(milliseconds to wait=u32 100) -> ()  [unwired: 1 out]
            n178 = disable-structure shown="Enabled" {
              disable-tunnel: [w189 w190] -> w179
              frame Enabled {
                n179 = property on="editSpeed" class="DigNum (strict)"() -> ("Value"=w189:dbl)  [unwired: 2 in, 2 out]
              }
              frame Disabled {
                n180 = property on="velocidade" class="DigNum (strict)"() -> ("Value"=w190:u32)  [unwired: 2 in, 2 out]
              }
            }
            n181 = property on="editSetLowerLimit" class="DigNum (strict)"() -> ("Value"=w181:u32)  [unwired: 2 in, 2 out]
            n182 = Less Or Equal?(x=w179, y=w181) -> (x <= y?=w185:bool)
            n183 = case shown="True" w185 {
              selector: w185 -> [w191 _]
              tunnel: [w191 w192] -> w183
              frame False {
              }
              frame True {
                n184 = flat-sequence {
                  tunnel: [w198] -> w193
                  tunnel: w193 -> [w202]
                  tunnel: [w201] -> w192
                  frame #0 {
                    n185 = local read "editCountLowerLimit"() -> (w197:u8)
                    n186 = Increment(x=w197) -> (x+1=w196:u8)
                    n187 = local write "editCountLowerLimit"(w196) -> ()
                    n188 = local read "editTotalLowerLimit"() -> (w195:u8)
                    n189 = Subtract(x=w195, y=w196) -> (x-y=w194:u8)
                    n190 = property on="slideWaitLowerTime" class="Slide (strict)"("Value"=w194) -> ()  [unwired: 2 in, 2 out]
                  }
                  frame #1 {
                    n191 = local read "editCountLowerLimit"() -> (w200:u8)
                    n192 = local read "editTotalLowerLimit"() -> (w199:u8)
                    n193 = Greater Or Equal?(x=w200, y=w199) -> (x >= y?=w198:bool)
                  }
                  frame #2 {
                    n194 = case shown="True" w202 {
                      selector: w202 -> [w203 w204]
                      tunnel: [w203 w204] -> w201
                      frame False {
                      }
                      frame True {
                        # "- Desliga o freio"
                        n195 = local write "ledBrake"(FALSE ("freio")) -> ()
                      }
                    }
                  }
                }
              }
            }
            n196 = Select(t=testMachine."wait " ("testMachine"), s=w183, f=testMachine."brake acquire" ("testMachine")) -> (s? t:f=w180:T2)
          }
          frame "exit" {
          }
          frame "wait " {
            # "- Aguarda 0.5s \n- Atualiza o numero de ciclos"
            n197 = flat-sequence {
              tunnel: [w219] -> w207
              frame #0 {
                n198 = local read "editCountWaitLimit"() -> (w215:u8)
                n199 = Increment(x=w215) -> (x+1=w216:u8)
                n200 = local write "editCountWaitLimit"(w216) -> ()
                n201 = local read "editTotalWaitLimit"() -> (w218:u8)
                n202 = Subtract(x=w218, y=w216) -> (x-y=w217:u8)
                n203 = property on="slideWaitTime" class="Slide (strict)"("Value"=w217) -> ()  [unwired: 2 in, 2 out]
              }
              frame #1 {
                n204 = local read "editCountWaitLimit"() -> (w221:u8)
                n205 = local read "editTotalWaitLimit"() -> (w220:u8)
                n206 = Greater Or Equal?(x=w221, y=w220) -> (x >= y?=w219:bool)
              }
            }
            n207 = disable-structure shown="Enabled" {
              frame Enabled {
                n208 = local read "ledWaitState"() -> (w228:bool)
                n209 = Not(x=w228) -> (.not. x?=w227:bool)
                n210 = local write "ledBrakeState"(FALSE ("ledBrakeState")) -> ()
                n211 = local write "ledWaitState"(w227) -> ()
              }
              frame Disabled {
              }
            }
            n212 = Wait (ms)(milliseconds to wait=u32 100) -> ()  [unwired: 1 out]
            n213 = case shown="True" w207 {
              selector: w207 -> [w222 _]
              tunnel: [w222 w226] -> w208
              frame False {
              }
              frame True {
                n214 = local read "editSetNumberOfCycles"() -> (w224:u16)
                n215 = local read "editCurrCycleCtr"() -> (w223:u32)
                n216 = Greater Or Equal?(x=w223, y=w224) -> (x >= y?=w226:bool)
                n217 = Not(x=w226) -> (.not. x?=w225:bool)
                n218 = local write "ledEnsaio"(w225) -> ()
              }
            }
            n219 = Select(t=testMachine."motor" ("testMachine"), s=w207, f=testMachine."wait " ("testMachine")) -> (s? t:f=w209:T2)
            n220 = Select(t=testMachine."finish" ("testMachine"), s=w208, f=w209) -> (s? t:f=w213:T2)
          }
        }
        n221 = disable-structure shown="Enabled" {
          frame Disabled {
          }
          frame Enabled {
            n222 = local write "ledReadyState"(FALSE ("ledReady")) -> ()
            n223 = local write "ledRunningState"(TRUE ("ledReady")) -> ()
          }
        }
        n224 = local read "buttonStart"() -> (w84:bool)
        n225 = Select(t=mainMachine."running" ("mainMachine"), s=w84, f=mainMachine."blocked" ("mainMachine")) -> (s? t:f=w81:T1)
      }
      frame "blocked" {
        n226 = local read "buttonStart"() -> (w234:bool)
        n227 = Select(t=mainMachine."ready" ("mainMachine"), s=w234, f=mainMachine."blocked" ("mainMachine")) -> (s? t:f=w230:T1)
        n228 = local write "ledRunningState"(FALSE ("ledReady")) -> ()
        n229 = local write "ledBlockState"(TRUE ("ledReady")) -> ()
      }
      frame "finish" {
        n230 = local write "ledBlockState"(FALSE ("ledReady")) -> ()
      }
    }
    "mainMachine" <- w11
    "testMachine" <- w12
  }
  n231 = while {
    tunnel: "stop" -> [w247]
    stop <- w247 stop-if-true
    n232 = local read "ledInit2State"() -> (w242:bool)
    n233 = local read "ledEnsaio"() -> (w240:bool)
    n234 = Wait Until Next ms Multiple(millisecond multiple=u32 10) -> ()  [unwired: 1 out]
    n235 = call "Chronometer.vi"("start"=w240, "reset"=w242) -> ("Time"=w246:dbl)
    n236 = case shown="False" w240 {
      frame False {
      }
      frame True {
        n237 = local read "editSpeed"() -> (w250:dbl)
        n238 = Divide(x=w250, y=3.6) -> (x/y=w248:dbl)
        n239 = Multiply(x=w248, y=0.01) -> ()  [unwired: 1 out]
      }
    }
    n240 = Format Date/Time String(time format string (%c)="%H:%M:%S", seconds (now)=w246, UTC format=TRUE) -> (date/time string=w243:string)
    n241 = local write "labelTestTime"(w243) -> ()
  }
  n242 = while {
    tunnel: "stop" -> [w256]
    tunnel: w3 -> [w254]
    tunnel: w2 -> [w253]
    stop <- w256 stop-if-true
    n243 = local read "ledEnsaio"() -> (w252:bool)
    n244 = case shown="True" w252 {
      tunnel: w256 -> [_ w259]
      tunnel: w252 -> [_ w268]
      tunnel: w254 -> [w258 w263]
      tunnel: w253 -> [w257 w262]
      tunnel: [w258 w261] -> _
      tunnel: [w257 w260] -> _
      frame False {
      }
      frame True {
        n245 = while {
          tunnel: w263 -> [w297]
          tunnel: w262 -> [w296]
          tunnel: [w295] -> w261
          tunnel: [w294] -> w260
          tunnel: w259 -> [w293]
          stop <- w293 stop-if-true
          n246 = local read "ledRunningState"() -> (w291:bool)
          n247 = case shown="True" w291 {
            tunnel: w297 -> [w299 w342]
            tunnel: w296 -> [w298 w341]
            tunnel: [w299 w338] -> w295
            tunnel: [w298 w337] -> w294
            frame False {
            }
            frame True {
              w312 = 500.0
              w331 = 1000.0
              w356 = 1000.0
              w359 = 200.0
              n248 = VISA Write(VISA resource name=w342, write buffer="!", error in (no error)=w341) -> (VISA resource name out=w346:refnum<visa-resource-name>, error out=w345:errorcluster)  [unwired: 1 out]
              n249 = local read "editOffsetForce"() -> (w307:dbl)
              n250 = local read "editSetForce"() -> (w305:dbl)
              n251 = local read "editSetTempRefA"() -> (w334:dbl)
              n252 = local read "editSetTempRefB"() -> (w325:dbl)
              n253 = property class="Instr"(reference=w346, error in=w345) -> (reference out=w349:refnum<visa-resource-name>, error out=w348:errorcluster, "Bytes at Port"=w347:u32)
              n254 = VISA Read(VISA resource name=w349, byte count=w347, error in (no error)=w348) -> (VISA resource name out=w340:refnum<visa-resource-name>, read buffer=w343:string, error out=w339:errorcluster)  [unwired: 1 out]
              n255 = call "StringSplitter.vi"("Input String"=w343) -> ("S0"=w360:dbl, "S1"=w350:dbl, "S2"=w323:dbl, "S3"=w308:dbl)  [unwired: 11 in, 4 out]
              n256 = call "AnalogToMiliVolts.vi"("Input"=w308) -> ("Output"=w302:dbl)  [unwired: 10 in]
              n257 = call "AnalogToMiliVolts.vi"("Input"=w360) -> ("Output"=w313:dbl)  [unwired: 10 in]
              n258 = call "AnalogToMiliVolts.vi"("Input"=w323) -> ("Output"=w327:dbl)  [unwired: 10 in]
              n259 = call "AnalogToMiliVolts.vi"("Input"=w350) -> ("Output"=w351:dbl)  [unwired: 10 in]
              n260 = Subtract(x=w313, y=825.0) -> (x-y=w322:dbl)
              n261 = Divide(x=w302, y=w305) -> (x/y=w306:dbl)
              n262 = Multiply(x=w327, y=0.2) -> (x*y=w328:dbl)
              n263 = Multiply(x=w351, y=0.2) -> (x*y=w352:dbl)
              n264 = Divide(x=w322, y=15.0) -> (x/y=w319:dbl)
              n265 = Add(x=w306, y=w307) -> (x+y=w309:dbl)
              n266 = Add(x=w328, y=w325) -> (x+y=w329:dbl)
              n267 = Add(x=w352, y=w334) -> (x+y=w353:dbl)
              n268 = call "BoundaryLimits.vi"("UpperLimit"=w312, "UpperValue"=w312, "Input"=w309, "LowerLimit"=1.0, "LowerValue"=0.0) -> ("Output"=w303:dbl)
              n269 = call "BoundaryLimits.vi"("UpperLimit"=w359, "UpperValue"=w359, "Input"=w319, "LowerLimit"=1.0, "LowerValue"=0.0) -> ("Output"=w318:dbl)
              n270 = call "BoundaryLimits.vi"("UpperLimit"=w331, "UpperValue"=w331, "Input"=w329, "LowerLimit"=1.0, "LowerValue"=0.0) -> ("Output"=w324:dbl)
              n271 = call "BoundaryLimits.vi"("UpperLimit"=w356, "UpperValue"=w356, "Input"=w353, "LowerLimit"=1.0, "LowerValue"=0.0) -> ("Output"=w332:dbl)
              n272 = local read "editSpeedOffset"() -> (w316:dbl)
              n273 = local read "editSetSpeed"() -> (w317:dbl)
              n274 = local write "editForce"(w303) -> ()
              n275 = local write "graphForce"(w303) -> ()
              n276 = local write "editTempB"(w324) -> ()
              n277 = local write "editTempA"(w332) -> ()
              n278 = local write "editEngineSpeed"(w318) -> ()
              n279 = Multiply(x=w318, y=w317) -> (x*y=w315:dbl)
              n280 = Add(x=w315, y=w316) -> (x+y=w314:dbl)
              n281 = local write "graphSpeed"(w318) -> ()
              n282 = local write "editSpeed"(w314) -> ()
              n283 = disable-structure shown="Enabled" {
                frame Enabled {
                  n284 = property on="editSpeed" class="DigNum (strict)"() -> ("Value"=w361:dbl)  [unwired: 2 in, 2 out]
                  n285 = property on="editSpeed" class="DigNum (strict)"("Val(Sgnl)"=w361) -> ()  [unwired: 2 in, 2 out]
                }
                frame Disabled {
                  n286 = property on="velocidade 2" class="DigNum (strict)"() -> ("Value"=w362:u32)  [unwired: 2 in, 2 out]
                  n287 = property on="velocidade" class="DigNum (strict)"("Val(Sgnl)"=w362) -> ()  [unwired: 2 in, 2 out]
                }
              }
              n288 = local read "ledBrake"() -> (w301:bool)
              n289 = local read "ledMotor"() -> (w300:bool)
              n290 = call "DigitalToString.vi"("D3"=FALSE, "D2"=w300, "D1"=w301) -> ("String"=w336:string)  [unwired: 1 out]
              n291 = VISA Write(VISA resource name=w340, write buffer=w336, error in (no error)=w339) -> (VISA resource name out=w338:refnum<visa-resource-name>, error out=w337:errorcluster)  [unwired: 1 out]
            }
          }
          n292 = Wait (ms)(milliseconds to wait=u32 200) -> ()  [unwired: 1 out]
        }
        n293 = local read "editSetPathToFile"() -> (w270:path)
        n294 = local read "editEngineSpeed"() -> (w266:dbl)
        n295 = local read "editSpeed"() -> (w267:dbl)
        n296 = local read "editSpeed"() -> (w264:dbl)
        n297 = local read "editTempA"() -> (w282:dbl)
        n298 = local read "editForce"() -> (w265:dbl)
        n299 = Path To String(path=w270) -> (string=w269:string)
        n300 = call "Convert to Dynamic Data9"("Double"=w266) -> ("Dynamic Data Type"=w286:dynamicdata)  [unwired: 3 in]
        n301 = call "Convert to Dynamic Data10"("Double"=w267) -> ("Dynamic Data Type"=w287:dynamicdata)  [unwired: 3 in]
        n302 = call "Convert to Dynamic Data6"("Double"=w282) -> ("Dynamic Data Type"=w283:dynamicdata)  [unwired: 3 in]
        n303 = call "Convert to Dynamic Data7"("Double"=w265) -> ("Dynamic Data Type"=w284:dynamicdata)  [unwired: 3 in]
        n304 = call "Convert to Dynamic Data8"("Double"=w264) -> ("Dynamic Data Type"=w285:dynamicdata)  [unwired: 3 in]
        n305 = Concatenate Strings(w269, "\\data.lvm" ("string")) -> (w272:string)
        n306 = String To Path(string=w272) -> (path=w273:path)
        n307 = Merge Signals(w283, w284, w285, w286, w287) -> (w288:dynamicdata)
        n308 = xnode ("Set Dynamic Data Attributes")("Signals In"=w288) -> ("Signals Out"=w274:dynamicdata, "error out"=w276:errorcluster)  [unwired: 4 in]
        n309 = xnode ("Set Dynamic Data Attributes")("Signals In"=w274, "error in"=w276) -> ("Signals Out"=w275:dynamicdata, "error out"=w277:errorcluster)  [unwired: 3 in]
        n310 = xnode ("Set Dynamic Data Attributes")("Signals In"=w275, "error in"=w277) -> ("Signals Out"=w289:dynamicdata, "error out"=w278:errorcluster)  [unwired: 3 in]
        n311 = xnode ("Set Dynamic Data Attributes")("Signals In"=w289, "error in"=w278) -> ("Signals Out"=w290:dynamicdata, "error out"=w279:errorcluster)  [unwired: 3 in]
        n312 = xnode ("Set Dynamic Data Attributes")("Signals In"=w290, "error in"=w279) -> ("Signals Out"=w280:dynamicdata, "error out"=w281:errorcluster)  [unwired: 3 in]
        n313 = call "Write To Measurement File2"("Signals"=w280, "Enable"=w268, "error in (no error)"=w281, "Filename"=w273) -> ()  [unwired: 13 in, 3 out]
      }
    }
    n314 = Wait (ms)(milliseconds to wait=u32 10) -> ()  [unwired: 1 out]
  }
  n315 = disable-structure shown="Disabled" {
    frame Disabled {
    }
    frame Enabled {
    }
  }
  "velocidade" <- "velocidade 2"
